vi "findNextAvailableDriveLetter.vi"(8 "error in (no error)":errorcluster) -> (0 "error out":errorcluster, 3 "Next Available Disk Letter":string)   [LabVIEW 2017, in "BuildWorker Interface.lvlib" / "BuildWorker Controller.lvclass"]
uses:
  BuildWorker Controller.lvclass
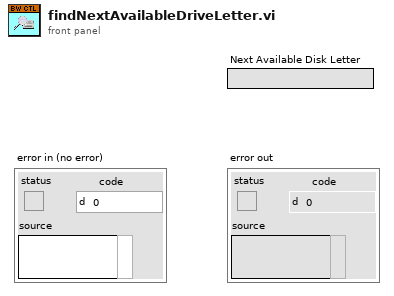
[diagram p1: front panel]
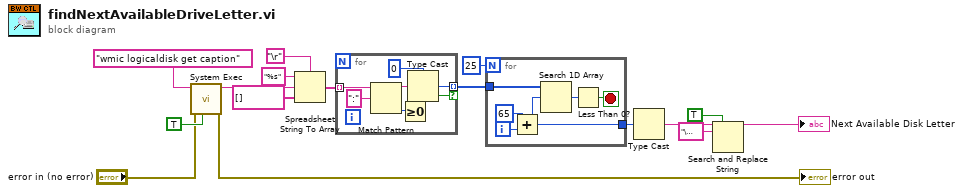
[diagram p0: block diagram]
diagram:
  n1 = call <vilib>:"System Exec.vi"("run minimized? (F)"=TRUE, "error in (no error)"="error in (no error)", "command line"="wmic logicaldisk get caption") -> ("error out"=→"error out":errorcluster, "standard output"=w12:string)  [unwired: 5 in, 2 out]
  n2 = Spreadsheet String To Array(delimiter (Tab)="\r", format string="%s", spreadsheet string=w12, array type (2D Dbl)=string[] []) -> (array=w11:string[])
  n3 = for {
    tunnel: w11 -> [w23] mode=indexing
    tunnel: [w18] -> w10 mode=indexing if=w20
    n4 = Match Pattern(string=w23, regular expression=":") -> (before substring=w19:string, offset past match=w21:i32)  [unwired: 1 in, 2 out]
    n5 = Greater Or Equal To 0?(x=w21) -> (x >= 0?=w20:bool)
    n6 = Type Cast(type=u8 0, x=w19) -> (*(type *) &x=w18:u8)
  }
  n7 = for {
    N: 25 -> [_]
    tunnel: w10 -> [w29]
    tunnel: [w24] -> w8
    i -> [w28]
    stop <- w25 stop-if-true
    n8 = Add(x=65, y=w28) -> (x+y=w24:i32)
    n9 = Search 1D Array(1D array=w29, element=w24) -> (index of element=w26:i32)  [unwired: 1 in]
    n10 = Less Than 0?(x=w26) -> (x < 0?=w25:bool)
  }
  n11 = Type Cast(x=w8) -> (*(type *) &x=w4:string)  [unwired: 1 in]
  n12 = Search and Replace String(replace all?=TRUE ("replace all? (F)"), input string=w4, search string="\u0000") -> (result string=→"Next Available Disk Letter":string)  [unwired: 5 in, 3 out]
